vi "built coordinate array.vi"(8 "error in (no error)":errorcluster, 9 "y coordinate":string, 10 "x coordinate":string, 11 "TomoConversion in":refnum<class "TomoConversion.lvclass">) -> (0 "error out":errorcluster, 3 "TomoConversion out":refnum<class "TomoConversion.lvclass">)   [LabVIEW 2012, in "TomoConversion.lvclass"]
uses:
  TomoConversion.lvclass
  TomoConversion.lvclass/TomoConversion.ctl
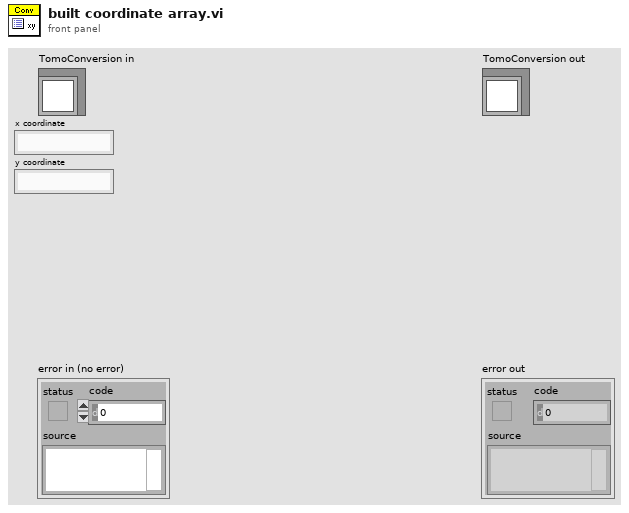
[diagram p1: front panel]
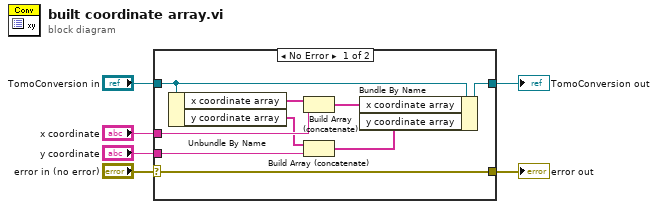
[diagram p0: block diagram]
diagram:
  n1 = case shown="No Error" "error in (no error)" {
    selector: "error in (no error)" -> [w15 w17]
    tunnel: [w15 w17] -> w5
    tunnel: [w13 w16] -> w3
    tunnel: "TomoConversion in" -> [w14 w16]
    tunnel: "x coordinate" -> [w11 _]
    tunnel: "y coordinate" -> [w7 _]
    frame No Error {
      n2 = Unbundle By Name(w14) -> ("x coordinate array"=w12:string[], "y coordinate array"=w8:string[])
      n3 = Build Array (concatenate)(w12, w11) -> (w10:string[])
      n4 = Build Array (concatenate)(w8, w7) -> (w9:string[])
      n5 = Bundle By Name(cluster=w14, "x coordinate array"=w10, "y coordinate array"=w9) -> (w13:refnum<class "TomoConversion.lvclass">)
    }
    frame Error {
    }
  }
  "error out" <- w5
  "TomoConversion out" <- w3
